vi "EvaluateFitCurves.vi"(0 "Zref":dbl=508.0 min=0.0, 1 "Fit Zmax":dbl, 2 "nPoints":i32, 3 "Fit Zmin":dbl, 5 "PowerLaw":cluster{"n":dbl, "d0":dbl}) -> (6 "PlotCluster":cluster{"Array":dbl[], "Array":dbl[]})   [LabVIEW 2013]
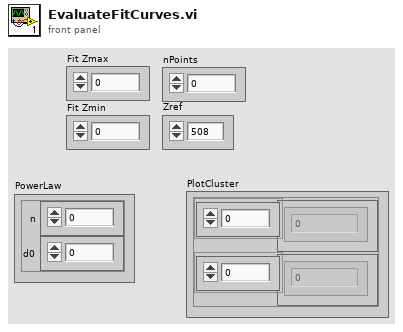
[diagram p1: front panel]
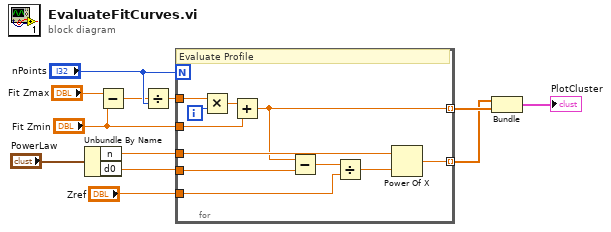
[diagram p0: block diagram]
diagram:
  n1 = Unbundle By Name("PowerLaw") -> ("n"=w6:dbl, "d0"=w5:dbl)
  n2 = Subtract(x="Fit Zmax", y="Fit Zmin") -> (x-y=w3:dbl)
  n3 = Divide(x=w3, y="nPoints") -> (x/y=w8:dbl)
  n4 = for {
    N: "nPoints" -> [_]
    tunnel: w8 -> [w23]
    tunnel: [w14] -> w11 mode=indexing
    tunnel: w5 -> [w20]
    tunnel: w6 -> [w19]
    tunnel: [w16] -> w10 mode=indexing
    tunnel: "Zref" -> [w15]
    tunnel: "Fit Zmin" -> [w13]
    i -> [w22]
    # "Evaluate Profile"
    n5 = Multiply(x=w23, y=w22) -> (x*y=w21:dbl)
    n6 = Add(x=w21, y=w13) -> (x+y=w14:dbl)
    n7 = Subtract(x=w14, y=w20) -> (x-y=w18:dbl)
    n8 = Divide(x=w18, y=w15) -> (x/y=w17:dbl)
    n9 = Power Of X(1:w17, 2:w19) -> (0:w16:dbl)
  }
  n10 = Bundle(w10, w11) -> (→"PlotCluster":cluster{dbl[], dbl[]})  [unwired: 1 in]
